vi "GetLastError.vi"(8 "Error In":errorcluster) -> (0 "error IO":errorcluster, 2 "Last Error":errorcluster)   [LabVIEW 2017, in "UserInterface.lvlib"]
uses:
  UserInterface.lvlib
  States_FGVQ.ctl
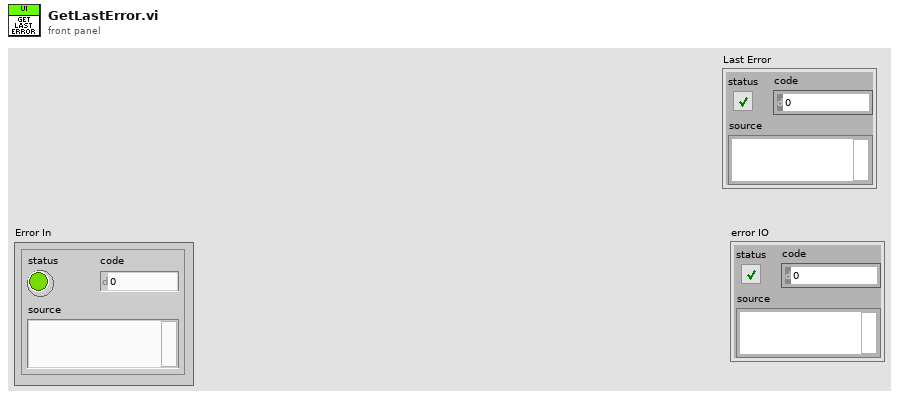
[diagram p1: front panel]
types:
  T1 = typedef "UserInterface.lvlib/States_FGVQ.ctl" = enum16{"Get", "Shutdown", "Initialize"}
  T2 = typedef "ErrorHandler.lvlib/MessageData.ctl" = cluster{"State":T3, "Payload":variant, "WaitOnReply":bool, "ReplyNotif":refnum<notifier>}
  T3 = typedef "ErrorHandler.lvlib/States_Module.ctl" = enum16{"DoSomething", "Shutdown", "Initialize"}
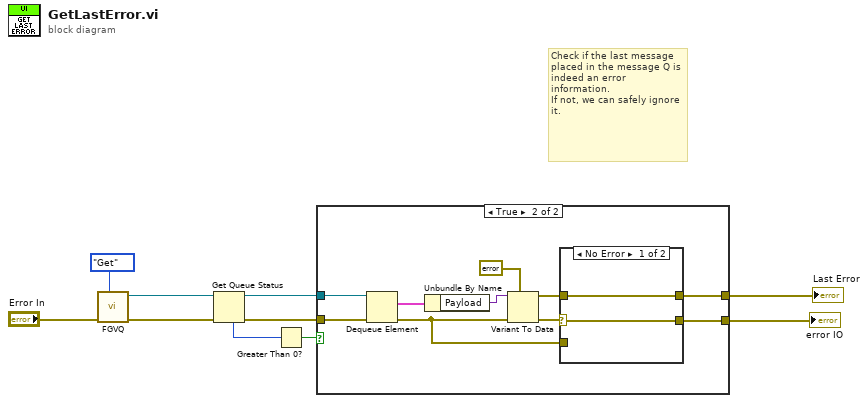
[diagram p0: block diagram]
diagram:
  # "Check if the last message \nplaced in the message Q is indeed an error information.\nIf not, we can safely ignore it."
  n1 = call "FGVQ.vi"("State"=States_FGVQ."Get", "Error In"="Error In") -> ("Error Out"=w8:errorcluster, "queue out"=w7:refnum<queue>)  [unwired: 8 in]
  n2 = Get Queue Status(queue=w7, error in (no error)=w8) -> (queue out=w3:refnum<queue>, error out=w4:errorcluster, # elements in queue=w6:i32)  [unwired: 1 in, 5 out]
  n3 = Greater Than 0?(x=w6) -> (x > 0?=w5:bool)
  n4 = case shown="True" w5 {
    tunnel: w4 -> [w11 w21]
    tunnel: w3 -> [_ w20]
    tunnel: [w11 w14] -> w2
    tunnel: [w11 w12] -> w1
    frame False {
    }
    frame True {
      n5 = Dequeue Element(queue=w20, error in (no error)=w21) -> (element=w19:T2, error out=w13:errorcluster)  [unwired: 1 in, 2 out]
      n6 = Unbundle By Name(w19) -> ("Payload"=w17:variant)
      n7 = Variant To Data(error in=w13, type=errorcluster {"status"=FALSE, "code"=0, "source"=""} ("Error Out"), Variant=w17) -> (data=w15:errorcluster, error out=w16:errorcluster)
      n8 = case shown="No Error" w16 {
        selector: w16 -> [w23 _]
        tunnel: w15 -> [w22 _]
        tunnel: [w23 w24] -> w14
        tunnel: w13 -> [_ w24]
        tunnel: [w22 w24] -> w12
        frame No Error {
        }
        frame Error {
        }
      }
    }
  }
  "error IO" <- w2
  "Last Error" <- w1
